vi "Read Cuenta.vi"(11 "Hijo in":refnum<class "Hijo.lvclass">) -> (2 "Cuenta":dbl, 3 "Hijo out":refnum<class "Hijo.lvclass">)   [LabVIEW 2020, in "Hijo.lvlib" / "Hijo.lvclass"]
uses:
  Hijo.lvclass
  Hijo.lvclass/Hijo.ctl
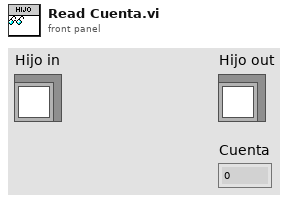
[diagram p1: front panel]
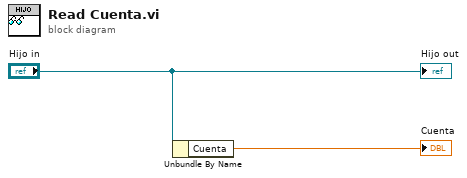
[diagram p0: block diagram]
diagram:
  n1 = Unbundle By Name("Hijo in") -> ("Cuenta"=→"Cuenta":dbl)
  "Hijo out" <- "Hijo in"
